vi "ButtonPress.vi"(1 "Input":bool) -> (0 "Output":bool)   [LabVIEW 2017]
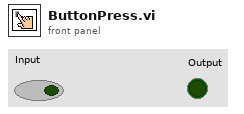
[diagram p1: front panel]
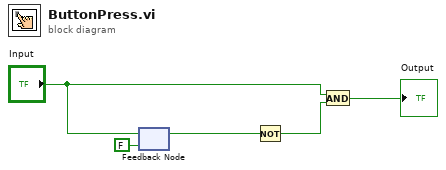
[diagram p0: block diagram]
diagram:
  n1 = feedback-in #1("Input") -> ()
  n2 = feedback #1(FALSE ("Input")) -> (w3:bool)
  n3 = Not(x=w3) -> (.not. x?=w4:bool)
  n4 = And(x="Input", y=w4) -> (x .and. y?=→"Output":bool)
